vi "Read Engine DataSet.vi"(8 "error in (no error)":errorcluster, 11 "HW Engine in":refnum<class "HW Engine.lvclass">) -> (0 "error out":errorcluster, 2 "Engine DataSet":string[][](array[string]), 3 "HW Engine out":refnum<class "HW Engine.lvclass">)   [LabVIEW 2025]
uses:
  HW Engine.lvclass
  HW Engine.lvclass/HW Engine.ctl
  C:/Users/Public/Documents/Sandia National Labs/TSS Plugin/CEF.lvlibp/serializable node/CEF_serializable node.lvclass
  C:/Users/Public/Documents/Sandia National Labs/TSS Plugin/CEF.lvlibp/Node/CEF_Node.lvclass
  C:/Working copy/tss/Plugin/HW Engine/HW Engine/HW Engine.lvclass
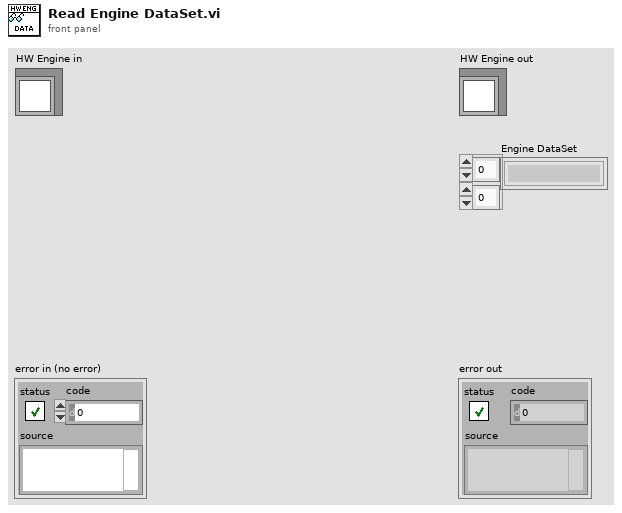
[diagram p1: front panel]
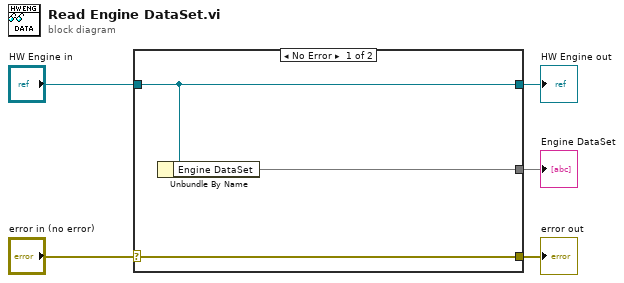
[diagram p0: block diagram]
diagram:
  n1 = case shown="No Error" "error in (no error)" {
    selector: "error in (no error)" -> [w8 w9]
    tunnel: [w8 w9] -> w4
    tunnel: [w7 w10] -> w2
    tunnel: "HW Engine in" -> [w7 w10]
    tunnel: [w6 _] -> w1
    frame No Error {
      n2 = Unbundle By Name(w7) -> ("Engine DataSet"=w6)
    }
    frame Error {
    }
  }
  "error out" <- w4
  "HW Engine out" <- w2
  "Engine DataSet" <- w1
